vi "editScriptCommandLimits.vi"() -> ()   [LabVIEW 2015]
doc: "Use this template to build a producer/consumer design pattern with events to produce queue items. Use this design pattern instead of the User Interface Event Handler pattern for user interfaces when you want to execute code asynchronously in response to an event without slowing the user interface responsiveness."
panel:
  out "Script Command":string
  in  "Back Up before saving":bool
  in  "Enter Line Number":u32
  in  "Save Line":bool
  in  "stop":bool
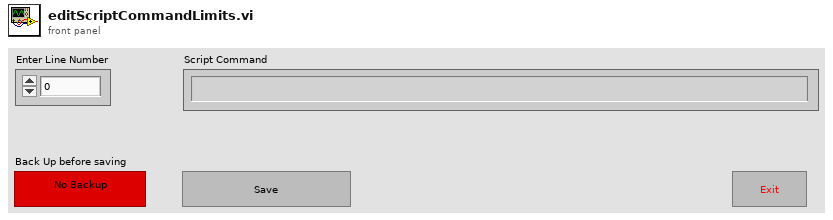
[diagram p1: front panel]
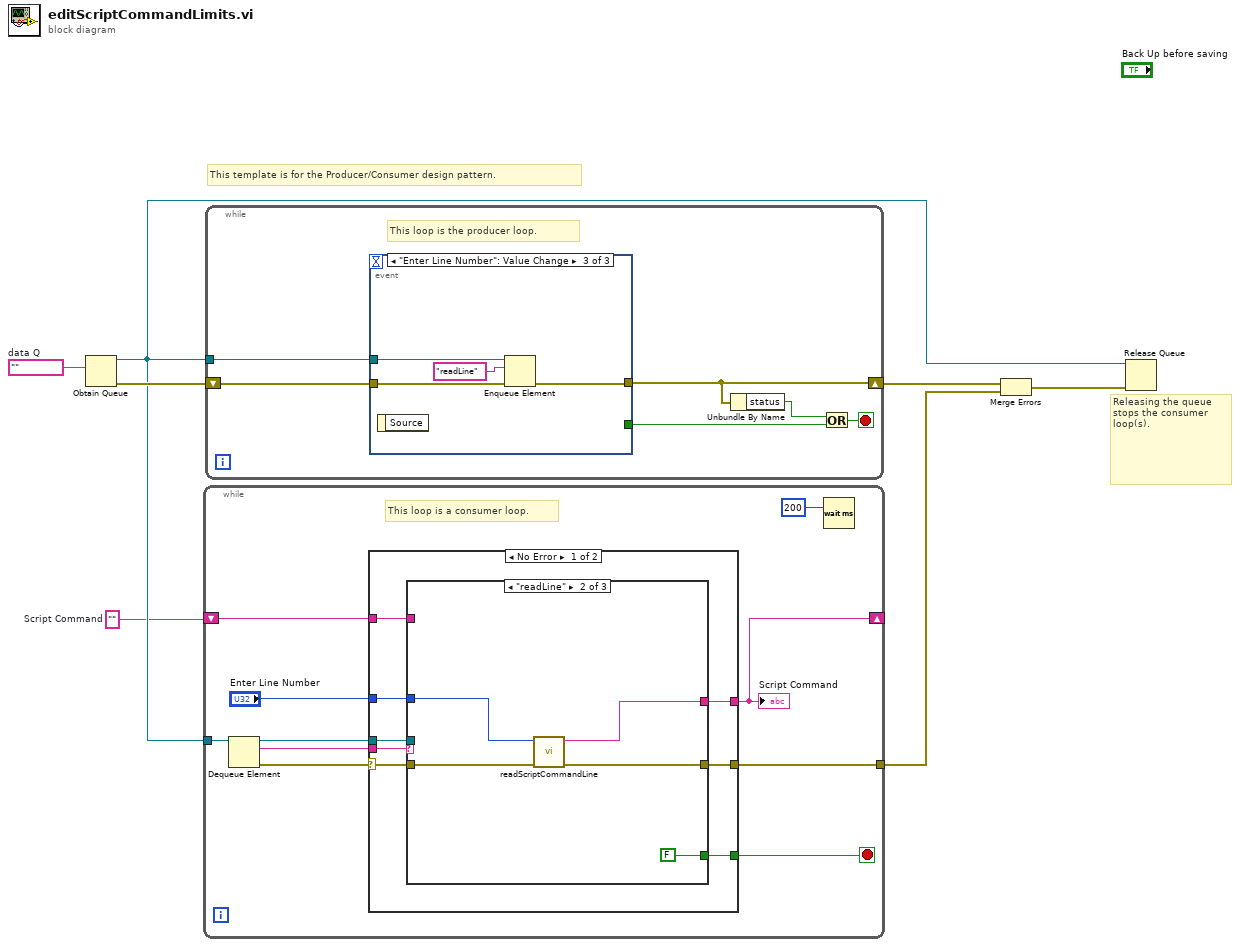
[diagram p0: block diagram]
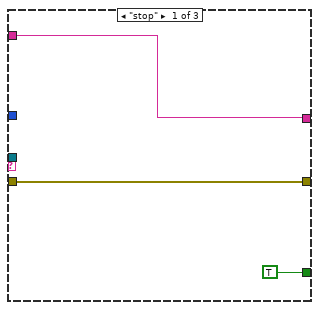
[diagram p2: hidden frame]
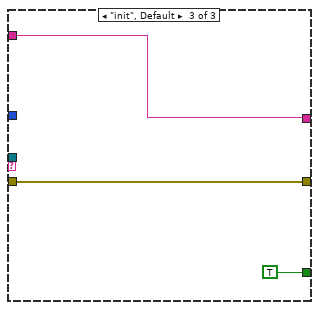
[diagram p3: hidden frame]
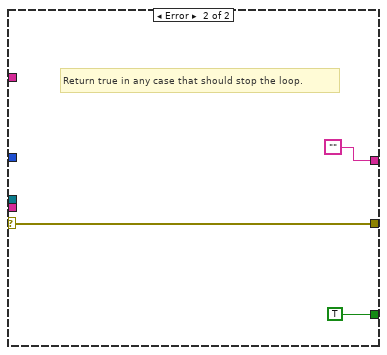
[diagram p4: hidden frame]
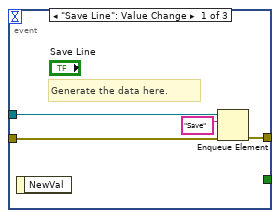
[diagram p5: hidden frame]
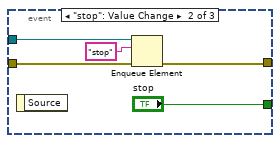
[diagram p6: hidden frame]
diagram:
  w1 = ""  # Script Command
  w5 = ""  # data Q
  # "Releasing the queue stops the consumer loop(s)."
  # "This template is for the Producer/Consumer design pattern."
  n1 = Obtain Queue(element data type=w5) -> (queue out=w4:refnum<queue>, error out=w7:errorcluster)  [unwired: 4 in, 1 out]
  n2 = while {
    tunnel: w4 -> [w17]
    tunnel: [w13] -> w2
    shift-right: [w10] -> _
    shift-left: w1 -> [w9]
    stop <- w14 stop-if-true
    # "This loop is a consumer loop."
    n3 = Dequeue Element(queue=w17) -> (queue out=w12:refnum<queue>, element=w15:string, error out=w16:errorcluster)  [unwired: 2 in, 1 out]
    n4 = case shown="No Error" w16 {
      selector: w16 -> [w23 w38]
      tunnel: w15 -> [w21 _]
      tunnel: [w25 TRUE] -> w14
      tunnel: [w22 w38] -> w13
      tunnel: w12 -> [w24 _]
      tunnel: [w20 ""] -> w10
      tunnel: w9 -> [w19 _]
      tunnel: "Enter Line Number" -> [w18 _]
      frame No Error {
        n5 = case shown="\"readLine\"" w21 {
          tunnel: [TRUE FALSE TRUE] -> w25
          tunnel: w24 -> [_ _ _]
          tunnel: w23 -> [w27 w32 w35]
          tunnel: [w27 w31 w35] -> w22
          tunnel: [w26 w30 w34] -> w20
          tunnel: w19 -> [w26 _ w34]
          tunnel: w18 -> [_ w29 _]
          frame "stop" {
          }
          frame "readLine" {
            n6 = call "readScriptCommandLine.vi"("error in (no error)"=w32, "Enter Line Number"=w29) -> ("error out"=w31:errorcluster, "standard output"=w30:string)  [unwired: 8 in]
          }
          frame "init", Default {
          }
        }
      }
      frame Error {
        # "Return true in any case that should stop the loop."
      }
    }
    "Script Command" <- w10
    n7 = Wait (ms)(milliseconds to wait=u32 200) -> ()  [unwired: 1 out]
  }
  n8 = while {
    shift-right: [w41] -> w6
    shift-left: w7 -> [w44]
    tunnel: w4 -> [w45]
    stop <- w42 stop-if-true
    # "This loop is the producer loop."
    n9 = event shown="[2] \"Enter Line Number\": Value Change" {
      selector: _ -> [_ _ _]
      dyn-events: _ -> [_ _ _]
      timeout: _ -> [_ _ _]
      tunnel: w45 -> [w49 w50 w55]
      tunnel: w44 -> [w48 w52 w56]
      tunnel: [w47 w51 w57] -> w41
      tunnel: [_ "stop" _] -> w43
      event "Save Line": Value Change {
        # "Generate the data here."
        n10 = event-data() -> ()  [unwired: 1 in, 1 out]
        n11 = Enqueue Element(queue=w49, element="Save", error in (no error)=w48) -> (error out=w47:errorcluster)  [unwired: 1 in, 2 out]
      }
      event "stop": Value Change {
        n12 = event-data() -> ()  [unwired: 1 in, 1 out]
        n13 = Enqueue Element(queue=w50, element="stop", error in (no error)=w52) -> (error out=w51:errorcluster)  [unwired: 1 in, 2 out]
      }
      event "Enter Line Number": Value Change {
        n14 = event-data() -> ()  [unwired: 1 in, 1 out]
        n15 = Enqueue Element(queue=w55, element="readLine", error in (no error)=w56) -> (error out=w57:errorcluster)  [unwired: 1 in, 2 out]
      }
    }
    n16 = Unbundle By Name(w41) -> ("status"=w40:bool)
    n17 = Or(x=w40, y=w43) -> (x .or. y?=w42:bool)
  }
  n18 = Merge Errors(w6, w2) -> (w3:errorcluster)
  n19 = Release Queue(queue=w4, error in (no error)=w3) -> ()  [unwired: 1 in, 3 out]
